vi "PrepTip.vi"() -> ()   [LabVIEW 2014]
uses:
  <userlib>/Nanonis Prog Interface V5/Nanonis Prog Interface.lvlib
panel:
  in  "Pulse bias (V) (1)":dbl=1.0
  in  "Pulse width (s) (100m)":dbl=0.1 min=0.0 max=100.0 format="%#_6p"
  in  "y":i32
  in  "stop":bool
  in  "X (m)":sgl format="%.3p"
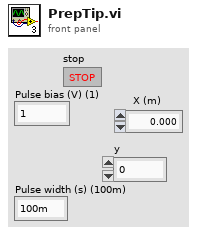
[diagram p1: front panel]
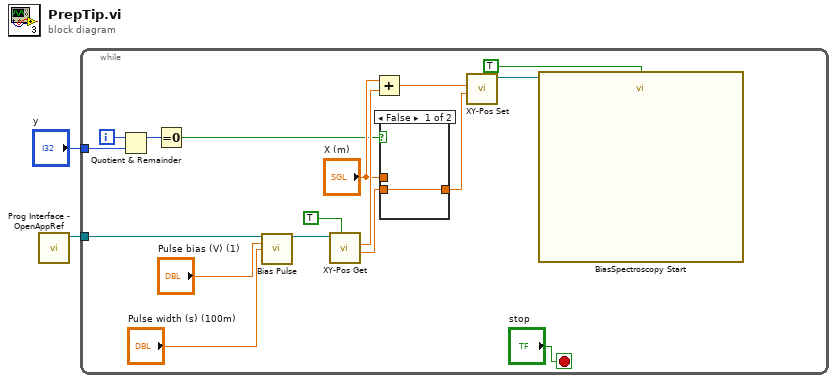
[diagram p0: block diagram]
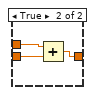
[diagram p2: hidden frame]
diagram:
  n1 = call <userlib>:"Prog Interface - OpenAppRef.vi"() -> ("Application reference"=w2:refnum<vi>)  [unwired: 6 in, 1 out]
  n2 = while {
    tunnel: w2 -> [w13]
    tunnel: "y" -> [w10]
    i -> [w11]
    stop <- "stop" stop-if-true
    n3 = Quotient & Remainder(x=w11, y=w10) -> (x-y*floor(x/y)=w9:i32)  [unwired: 1 out]
    n4 = Equal To 0?(x=w9) -> (x = 0?=w6:bool)
    n5 = call <userlib>:"Bias Pulse.vi"("Application ref in"=w13, "Pulse bias (V) (1)"="Pulse bias (V) (1)", "Pulse width (s) (100m)"="Pulse width (s) (100m)") -> ("Application ref out"=w15:refnum<vi>)  [unwired: 11 in, 1 out]
    n6 = call <userlib>:"XY-Pos Get.vi"("Wait for newest data (F=False)"=TRUE, "Application ref in"=w15) -> ("Y (m)"=w16:sgl, "X (m)"=w18:sgl)  [unwired: 5 in, 2 out]
    n7 = Add(x="X (m)", y=w18) -> (x+y=w17:sgl)
    n8 = case shown="False" w6 {
      tunnel: w16 -> [w20 w23]
      tunnel: [w20 w22] -> w8
      tunnel: "X (m)" -> [_ w21]
      frame False {
      }
      frame True {
        n9 = Add(x=w21, y=w23) -> (x+y=w22:sgl)
      }
    }
    n10 = call <userlib>:"XY-Pos Set.vi"("Y (m)"=w8, "X (m)"=w17) -> ("Application ref out"=w14:refnum<vi>)  [unwired: 6 in, 1 out]
    n11 = call <userlib>:"BiasSpectroscopy Start.vi"("Application ref in"=w14, "Get data (F)"=TRUE) -> ()  [unwired: 9 in, 5 out]
  }
